vi "PV HLT5xx Special.vi"(7 "Adress of unit":u16=1 min=1 max=999 step=1, 8 "error in (no error)":errorcluster, 10 "PV HLT5xx Special - Cluster":T1={"Parameter"=0, "Parameter\nread only<->describe"=FALSE, "Anodenpotential Mass 2"=905, "Anodenpotential Mass 3"=610, "Anodenpotential Mass 4"=465, "Filament"=0, "Zero time [s]"=5} {"Zero time [s]" min=2 max=200 step=1; "Filament" items=["Emission off", "Kathode 1, Emission on", "Kathode 2, Emission on", "Emission on"]; "Anodenpotential Mass 4" min=390 max=520 step=1; "Anodenpotential Mass 3" min=510 max=610 step=1; "Anodenpotential Mass 2" min=785 max=995 step=1; "Parameter" items=[" Preamplifier voltage [mV] (read only)", " Anode voltage [V] (read only)", " Kathode voltage [V] (read only)", " Suppressor voltage [V] (read only)", " Anodenpotential Mass 2 [V]", " Anodenpotential Mass 3 [V]", " Anodenpotential Mass 4 [V]", " Filament", " Zero time [s]"]}, 11 "VISA session":refnum<visa-resource-name>) -> (0 "error out":errorcluster, 2 "response (data)":string, 3 "dup VISA session":refnum<visa-resource-name>)   [LabVIEW 2016, in "Pfeiffer Vacuum.lvlib"]
doc: "There are 9 parameters available, only one of which can be enabled at a time. \n\n0 - Preamplifier voltage [mV] (read only) - Para 618\n1 - Anode voltage [V] (read only) - Para 620\n2 - Kathode voltage [V] (read only) - Para 621\n3 - Suppressor voltage [V] (read only) - Para 622\n4 - Anodenpotential Mass 2 [V] - Para 631\n5 - Anodenpotential Mass 3 [V] - Para 632\n6 - Anodenpotential Mass 4 [V] - Para 633\n7 - Filament - Para 645\n8 - Zero time [s] - Para 646\n\nNote: The 5 controls right of this one will set the appropriate values for the selected parameter. Any settings for an parameter that is not selected will be ignored. If a value is out of range, it will be changed to either the upper or the lower limit of the range."
uses:
  Pfeiffer Vacuum.lvlib
  PV HLT5xx Special - Cluster.ctl
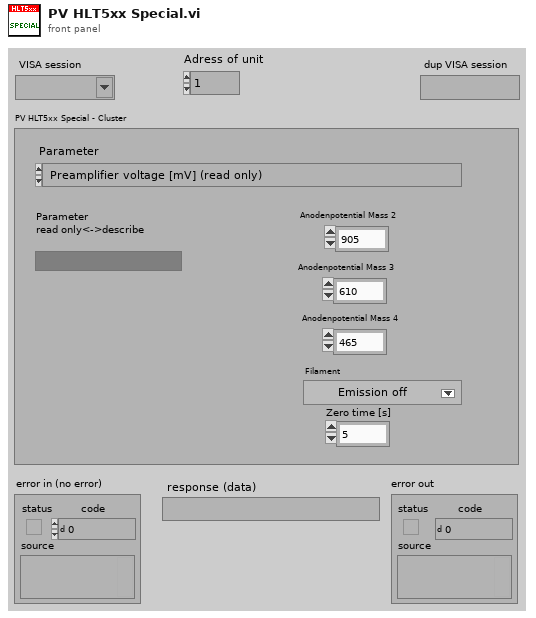
[diagram p1: front panel]
types:
  T1 = typedef "Pfeiffer Vacuum.lvlib/PV HLT5xx Special - Cluster.ctl" = cluster{"Parameter":u16, "Parameter\nread only<->describe":bool, "Anodenpotential Mass 2":u16, "Anodenpotential Mass 3":u16, "Anodenpotential Mass 4":u16, "Filament":u16, "Zero time [s]":u8}
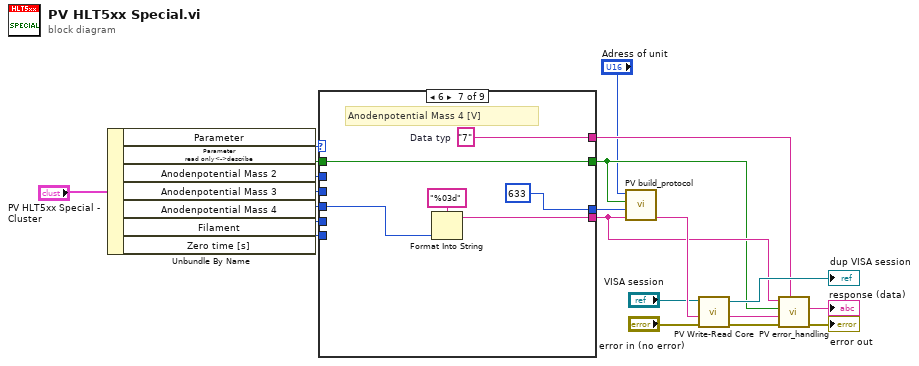
[diagram p0: block diagram]
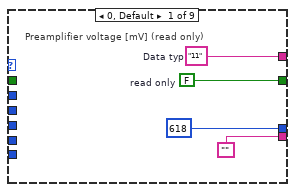
[diagram p2: hidden frame]
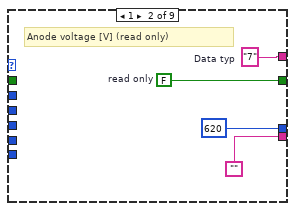
[diagram p3: hidden frame]
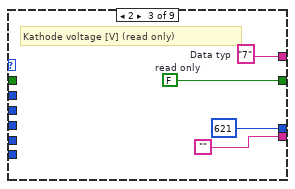
[diagram p4: hidden frame]
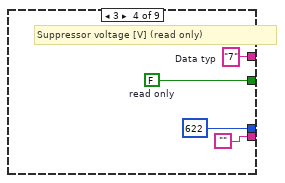
[diagram p5: hidden frame]
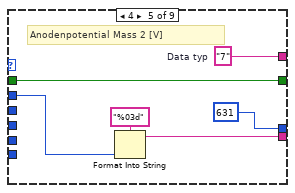
[diagram p6: hidden frame]
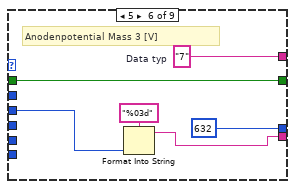
[diagram p7: hidden frame]
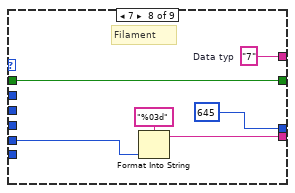
[diagram p8: hidden frame]
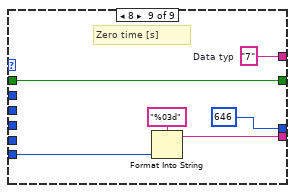
[diagram p9: hidden frame]
diagram:
  n1 = Unbundle By Name("PV HLT5xx Special - Cluster") -> ("Parameter"=w9:u16, "Parameter\nread only<->describe"=w20:bool, "Anodenpotential Mass 2"=w10:u16, "Anodenpotential Mass 3"=w7:u16, "Anodenpotential Mass 4"=w6:u16, "Filament"=w5:u16, "Zero time [s]"=w4:u8)
  n2 = case shown="6" w9 {
    tunnel: [u16 618 ("Parameter-number") u16 620 ("Parameter-number") u16 621 ("Parameter-number") u16 622 ("Parameter-number") u16 631 ("Parameter-number") u16 632 ("Parameter-number") u16 633 ("Parameter-number") u16 645 ("Parameter-number") u16 646 ("Parameter-number")] -> w21
    tunnel: ["" "" "" "" w38 w44 w50 w57 w63] -> w15
    tunnel: [w22 w27 w32 w36 w41 w47 w53 w59 w65] -> w13
    tunnel: w20 -> [_ _ _ _ w41 w47 w53 w59 w65]
    tunnel: [w25 w28 w30 w37 w43 w49 w55 w61 w67] -> w14
    tunnel: w10 -> [_ _ _ _ w39 _ _ _ _]
    tunnel: w7 -> [_ _ _ _ _ w45 _ _ _]
    tunnel: w6 -> [_ _ _ _ _ _ w51 _ _]
    tunnel: w5 -> [_ _ _ _ _ _ _ w56 _]
    tunnel: w4 -> [_ _ _ _ _ _ _ _ w62]
    frame 0, Default {
      w22 = FALSE  # read only
      w25 = "11"  # Data typ
      # "Preamplifier voltage [mV] (read only)"
    }
    frame 1 {
      w27 = FALSE  # read only
      w28 = "7"  # Data typ
      # "Anode voltage [V] (read only)"
    }
    frame 2 {
      w30 = "7"  # Data typ
      w32 = FALSE  # read only
      # "Kathode voltage [V] (read only)"
    }
    frame 3 {
      w36 = FALSE  # read only
      w37 = "7"  # Data typ
      # "Suppressor voltage [V] (read only)"
    }
    frame 4 {
      w43 = "7"  # Data typ
      # "Anodenpotential Mass 2 [V]"
      n3 = Format Into String(format string="%03d" ("Format-String"), w39) -> (resulting string=w38:string)  [unwired: 2 in, 1 out]
    }
    frame 5 {
      w49 = "7"  # Data typ
      # "Anodenpotential Mass 3 [V]"
      n4 = Format Into String(format string="%03d" ("Format-String"), w45) -> (resulting string=w44:string)  [unwired: 2 in, 1 out]
    }
    frame 6 {
      w55 = "7"  # Data typ
      # "Anodenpotential Mass 4 [V]"
      n5 = Format Into String(format string="%03d" ("Format-String"), w51) -> (resulting string=w50:string)  [unwired: 2 in, 1 out]
    }
    frame 7 {
      w61 = "7"  # Data typ
      # "Filament"
      n6 = Format Into String(format string="%03d" ("Format-String"), w56) -> (resulting string=w57:string)  [unwired: 2 in, 1 out]
    }
    frame 8 {
      w67 = "7"  # Data typ
      # "Zero time [s]"
      n7 = Format Into String(format string="%03d" ("Format-String"), w62) -> (resulting string=w63:string)  [unwired: 2 in, 1 out]
    }
  }
  n8 = call "PV build_protocol.vi"("Data"=w15, "Parameter-number"=w21, "parameter\nread<->describe"=w13, "Adress"="Adress of unit") -> ("output"=w19:string)  [unwired: 3 in]
  n9 = call "PV Write-Read Core.vi"("error in"="error in (no error)", "Write data in"=w19, "VISA session"="VISA session") -> ("error out"=w17:errorcluster, "response (data) out"=w18:string, "dup VISA session"=→"dup VISA session":refnum<visa-resource-name>)  [unwired: 2 in]
  n10 = call "PV error_handling.vi"("Data Typ in"=w14, "error in"=w17, "response (data) in"=w18, "Parameter\nread only<->describe"=w13, "data in"=w15) -> ("error out"=→"error out":errorcluster, "Data out"=→"response (data)":string)  [unwired: 4 in, 1 out]
